vi "Byte Buffer.Mapping.Write.vi"(8 "error in (no error)":errorcluster, 9 "initial buffer count (100)":i64=100, 10 "mappings":T1[](array[typedef]), 11 "Byte Buffer in":refnum<class "Byte Buffer.lvclass">) -> (0 "error out":errorcluster, 2 "mappings dup":T1[](array[typedef]), 3 "Byte Buffer out":refnum<class "Byte Buffer.lvclass">)   [LabVIEW 2016, in "VeriStand Data.lvlib" / "Byte Buffer.lvclass"]
uses:
  Byte Buffer.lvclass
  Byte Buffer.Mapping.ctl
  Typedefs/Typedefs.Data Types.ctl
  Byte Buffer.lvclass/Byte Buffer.ctl
  Byte Buffer.Write.vi
  Byte Buffer.Write (1D Boolean).vi
  Type Conversion/Type Conversion.From Double.Subset.vi
  Type Conversion/Type Conversion.From Double.Subset (1D Boolean).vi
  Byte Buffer.Write (1D SGL).vi
  Type Conversion/Type Conversion.From Double.Subset (1D SGL).vi
  Byte Buffer.Write (1D DBL).vi
  Byte Buffer.Write (1D I8).vi
  Type Conversion/Type Conversion.From Double.Subset (1D I8).vi
  Byte Buffer.Write (1D I16).vi
  Type Conversion/Type Conversion.From Double.Subset (1D I16).vi
  Byte Buffer.Write (1D I32).vi
  Type Conversion/Type Conversion.From Double.Subset (1D I32).vi
  Byte Buffer.Write (1D I64).vi
  Type Conversion/Type Conversion.From Double.Subset (1D I64).vi
  Byte Buffer.Write (1D U8).vi
  Type Conversion/Type Conversion.From Double.Subset (1D U8).vi
  Byte Buffer.Write (1D U16).vi
  Type Conversion/Type Conversion.From Double.Subset (1D U16).vi
  Byte Buffer.Write (1D U32).vi
  Type Conversion/Type Conversion.From Double.Subset (1D U32).vi
  Byte Buffer.Write (1D U64).vi
  Type Conversion/Type Conversion.From Double.Subset (1D U64).vi
  Byte Buffer.Write (String).vi
  Type Conversion/Type Conversion.From Double.vi
  Type Conversion/Type Conversion.From Double (1D Boolean).vi
  Type Conversion/Type Conversion.From Double (1D SGL).vi
  Type Conversion/Type Conversion.From Double (1D I8).vi
  Type Conversion/Type Conversion.From Double (1D I16).vi
  Type Conversion/Type Conversion.From Double (1D I32).vi
  Type Conversion/Type Conversion.From Double (1D I64).vi
  Type Conversion/Type Conversion.From Double (1D U8).vi
  Type Conversion/Type Conversion.From Double (1D U16).vi
  Type Conversion/Type Conversion.From Double (1D U32).vi
  Type Conversion/Type Conversion.From Double (1D U64).vi
  Byte Buffer.Buffer Subset.Set.vi
  Memory Management/Memory Management.MoveByteBlock.Read (String).vi
  Memory Management/Memory Management.Handle Return.vi
  VeriStand Data.lvlib
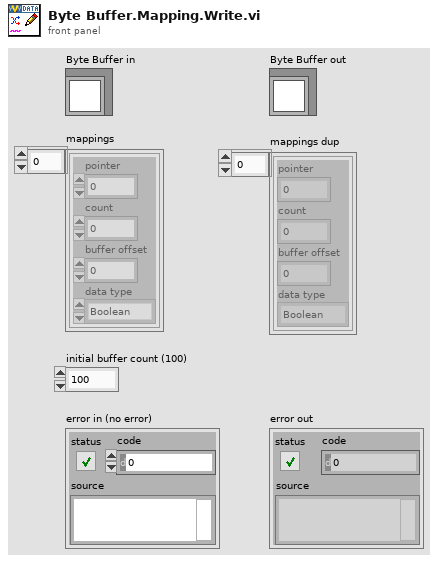
[diagram p1: front panel]
types:
  T1 = typedef "VeriStand Data.lvlib/Byte Buffer.lvclass/Byte Buffer.Mapping.ctl" = cluster{"pointer":u64, "count":i64, "buffer offset":u64, "data type":T2}
  T2 = typedef "VeriStand Data.lvlib/Typedefs.Data Types.ctl" = enum16{"Boolean", "Single", "Double", "I8", "I16", "I32", "I64", "U8", "U16", "U32", "U64"}
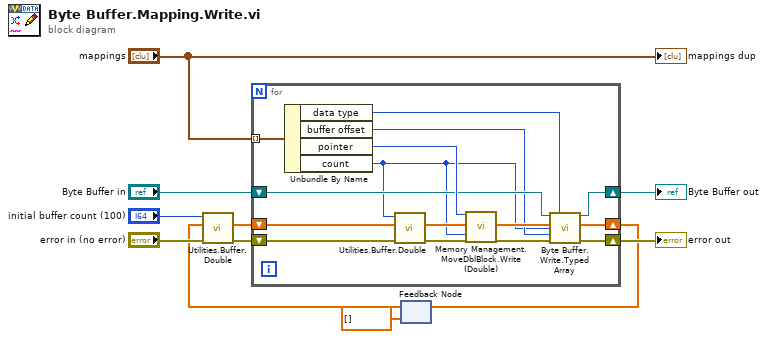
[diagram p0: block diagram]
diagram:
  n1 = feedback #1(dbl[] [] ("buffer out")) -> (w2:dbl[])
  n2 = call "Utilities.Buffer.Double.vi"("error in (no error)"="error in (no error)", "buffer in"=w2, "minimum size"="initial buffer count (100)") -> ("error out"=w5:errorcluster, "buffer out"=w3:dbl[])  [unwired: 7 in]
  n3 = for {
    tunnel: "mappings" -> [w26] mode=indexing
    shift-right: [w20] -> w11
    shift-left: w5 -> [w16]
    shift-right: [w23] -> w9
    shift-left: "Byte Buffer in" -> [w24]
    shift-right: [w17] -> w8
    shift-left: w3 -> [w15]
    n4 = Unbundle By Name(w26) -> ("data type"=w18:T2, "buffer offset"=w19:u64, "pointer"=w25:u64, "count"=w12:i64)
    n5 = call "Utilities.Buffer.Double.vi"("error in (no error)"=w16, "buffer in"=w15, "minimum size"=w12) -> ("error out"=w14:errorcluster, "buffer out"=w13:dbl[])  [unwired: 7 in]
    n6 = call "Memory Management.MoveDblBlock.Write (Double).vi"("src ptr in"=w25, "dst in"=w13, "count"=w12, "error in (no error)"=w14) -> ("dst out"=w22:dbl[], "error out"=w21:errorcluster)  [unwired: 10 in, 4 out]
    n7 = call "Byte Buffer.Write.Typed Array.vi"("Byte Buffer in"=w24, "data type"=w18, "buffer in"=w22, "count"=w12, "buffer offset"=w19, "error in (no error)"=w21) -> ("Byte Buffer out"=w23:refnum<class "Byte Buffer.lvclass">, "buffer out"=w17:dbl[], "error out"=w20:errorcluster)  [unwired: 6 in, 1 out]
  }
  "error out" <- w11
  "Byte Buffer out" <- w9
  n8 = feedback-in #1(w8) -> ()
  "mappings dup" <- "mappings"
